vi "FL_Make_data_frame_and_put_to_channel.vi"(8 "error in":errorcluster, 11 "VISA resource name in":refnum<visa-resource-name>) -> (0 "error out":errorcluster, 1 "High-speed channel":T1, 2 "Timestamp":timestamp, 3 "VISA resource name out":refnum<visa-resource-name>, 5 "Read buffer (for reference only, data is queued)":string)   [LabVIEW 2016]
uses:
  <extravilib>/ChannelInstances/High Speed Stream-c(str,stamp)/)Channel.ctl
  <extravilib>/ChannelInstances/High Speed Stream-c(str,stamp)/)Channel.vi
  <extravilib>/ChannelInstances/High Speed Stream-c(str,stamp).lvlib
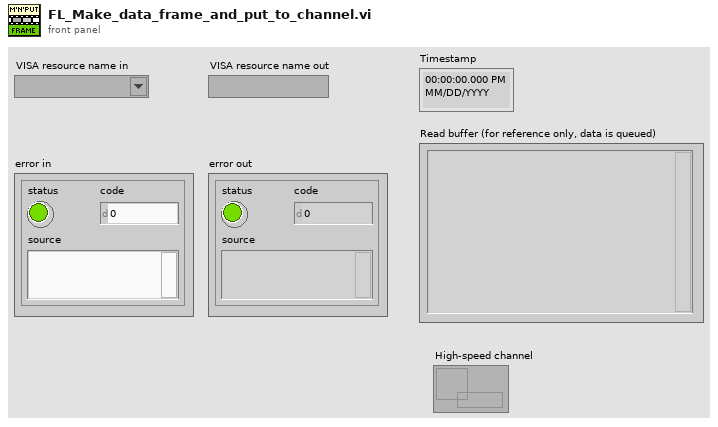
[diagram p1: front panel]
types:
  T1 = typedef "High Speed Stream-c(str,stamp).lvlib/)Channel.ctl" = refnum<queue>
  T2 = cluster{string, "seconds since 1Jan1904":timestamp}
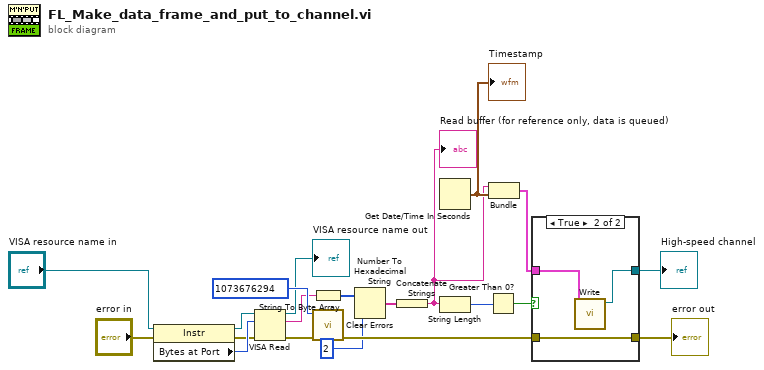
[diagram p0: block diagram]
diagram:
  n1 = property class="Instr"(reference="VISA resource name in", error in="error in") -> (reference out=w9:refnum<visa-resource-name>, error out=w10:errorcluster, "Bytes at Port"=w11:u32)
  n2 = VISA Read(VISA resource name=w9, byte count=w11, error in (no error)=w10) -> (VISA resource name out=→"VISA resource name out":refnum<visa-resource-name>, read buffer=w4:string, error out=w14:errorcluster)  [unwired: 1 out]
  n3 = String To Byte Array(string=w4) -> (unsigned byte array=w6:u8[])
  n4 = call <vilib>:"Clear Errors.vi"("error in (no error)"=w14, "specific error code to clear (0: all)"=1073676294) -> ("error out"=w17:errorcluster)  [unwired: 4 in, 1 out]
  n5 = Number To Hexadecimal String(1:i16 2 ("width (-)"), 2:w6) -> (0:w5:string[])
  n6 = Concatenate Strings(w5) -> (w3:string)
  "Read buffer (for reference only, data is queued)" <- w3
  n7 = Get Date/Time In Seconds ("Current time")() -> (seconds since 1Jan1904=w15:timestamp)
  "Timestamp" <- w15
  n8 = String Length(string=w3) -> (length=w19:i32)
  n9 = Greater Than 0?(x=w19) -> (x > 0?=w20:bool)
  n10 = Bundle(w3, "seconds since 1Jan1904"=w15) -> (w16:T2)  [unwired: 1 in]
  n11 = case shown="True" w20 {
    tunnel: w16 -> [_ w23]
    tunnel: w17 -> [w21 w24]
    tunnel: [w21 w24] -> w18
    tunnel: [_ w22] -> w1
    frame False {
    }
    frame True {
      n12 = call <extravilib>:"Write.vi"("element"=w23) -> ("channel"=w22:T1)  [unwired: 8 in, 2 out]
    }
  }
  "error out" <- w18
  "High-speed channel" <- w1
